vi "数据主动和反控发送.vi"() -> ()   [LabVIEW 2016, in "数据传输系统-04.lvlib"]
uses:
  <vilib>/ptbypt/NI_PtbyPt.lvlib
panel:
  in  "N个五分钟":u32
  out "QN":string
  out "元素":cluster{"命令编码CN":string, "QN":string}[](array[cluster])
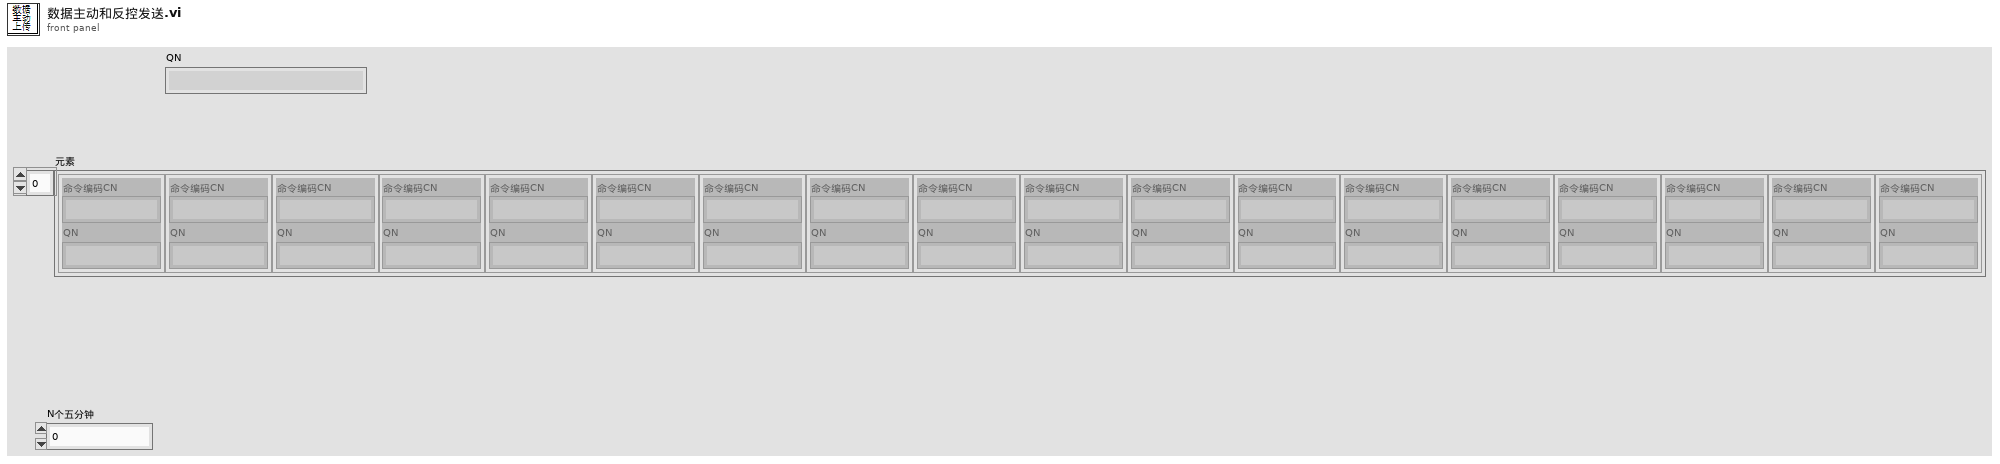
[diagram p1: front panel]
types:
  T1 = cluster{"setini":string, "sysini":string, "hechaini":string, "actualwrite":string, "actualread":string, "datasent":string, "反控命令信息队列":string, "反控与仪器交互":string}
  T2 = typedef "LVDateTimeRec.ctl" = cluster{"秒数的小数部分":dbl, "秒":i32, "分":i32, "时":i32, "日":i32, "月":i32, "年":i32, "天数（周）":i32, "天数（年）":i32, "DST":i32}
  T3 = enum16{"open", "replace", "create", "open or create", "replace or create", "replace or create with confirmation"}
  T4 = typedef "数据传输系统-04.lvlib/应用环境.ctl" = enum16{"STD", "GB212", "婉仪平台"}
  T5 = enum16{"关闭", "星期日", "星期一", "星期二", "星期三", "星期四", "星期五", "星期六"}
  T6 = enum16{"00点", "01点", "02点", "03点", "04点", "05点", "06点", "07点", "08点", "09点", "10点", "11点", "12点", "13点", "14点", "15点", "16点", "17点", "18点", "19点", "20点", "21点", "22点", "23点"}
  T7 = cluster{"[0]":string, "[1]":string, "[2]":string, "[3]":string, "[4]":string, "[5]":string, "[6]":string, "[7]":string, "[8]":string, "[9]":string, "[10]":string, "[11]":string, "[12]":string, "[13]":string, "[14]":string, "[15]":string, "[16]":string, "[17]":string, "[18]":string, "[19]":string, "[20]":string, "[21]":string, "[22]":string, "[23]":string, "[24]":string, "[25]":string, "[26]":string, "[27]":string, "[28]":string, "[29]":string, "[30]":string, "[31]":string, "[32]":string, "[33]":string, "[34]":string, "[35]":string, "[36]":string, "[37]":string, "[38]":string, "[39]":string, "[40]":string, "[41]":string, "[42]":string, "[43]":string, "[44]":string, "[45]":string, "[46]":string, "[47]":string, "[48]":string, "[49]":string, "[50]":string, "[51]":string, "[52]":string, "[53]":string, "[54]":string, "[55]":string, "[56]":string, "[57]":string, "[58]":string, "[59]":string, "[60]":string, "[61]":string, "[62]":string, "[63]":string, "[64]":string, "[65]":string, "[66]":string, "[67]":string, "[68]":string, "[69]":string, "[70]":string, "[71]":string, "[72]":string, "[73]":string, "[74]":string, "[75]":string}
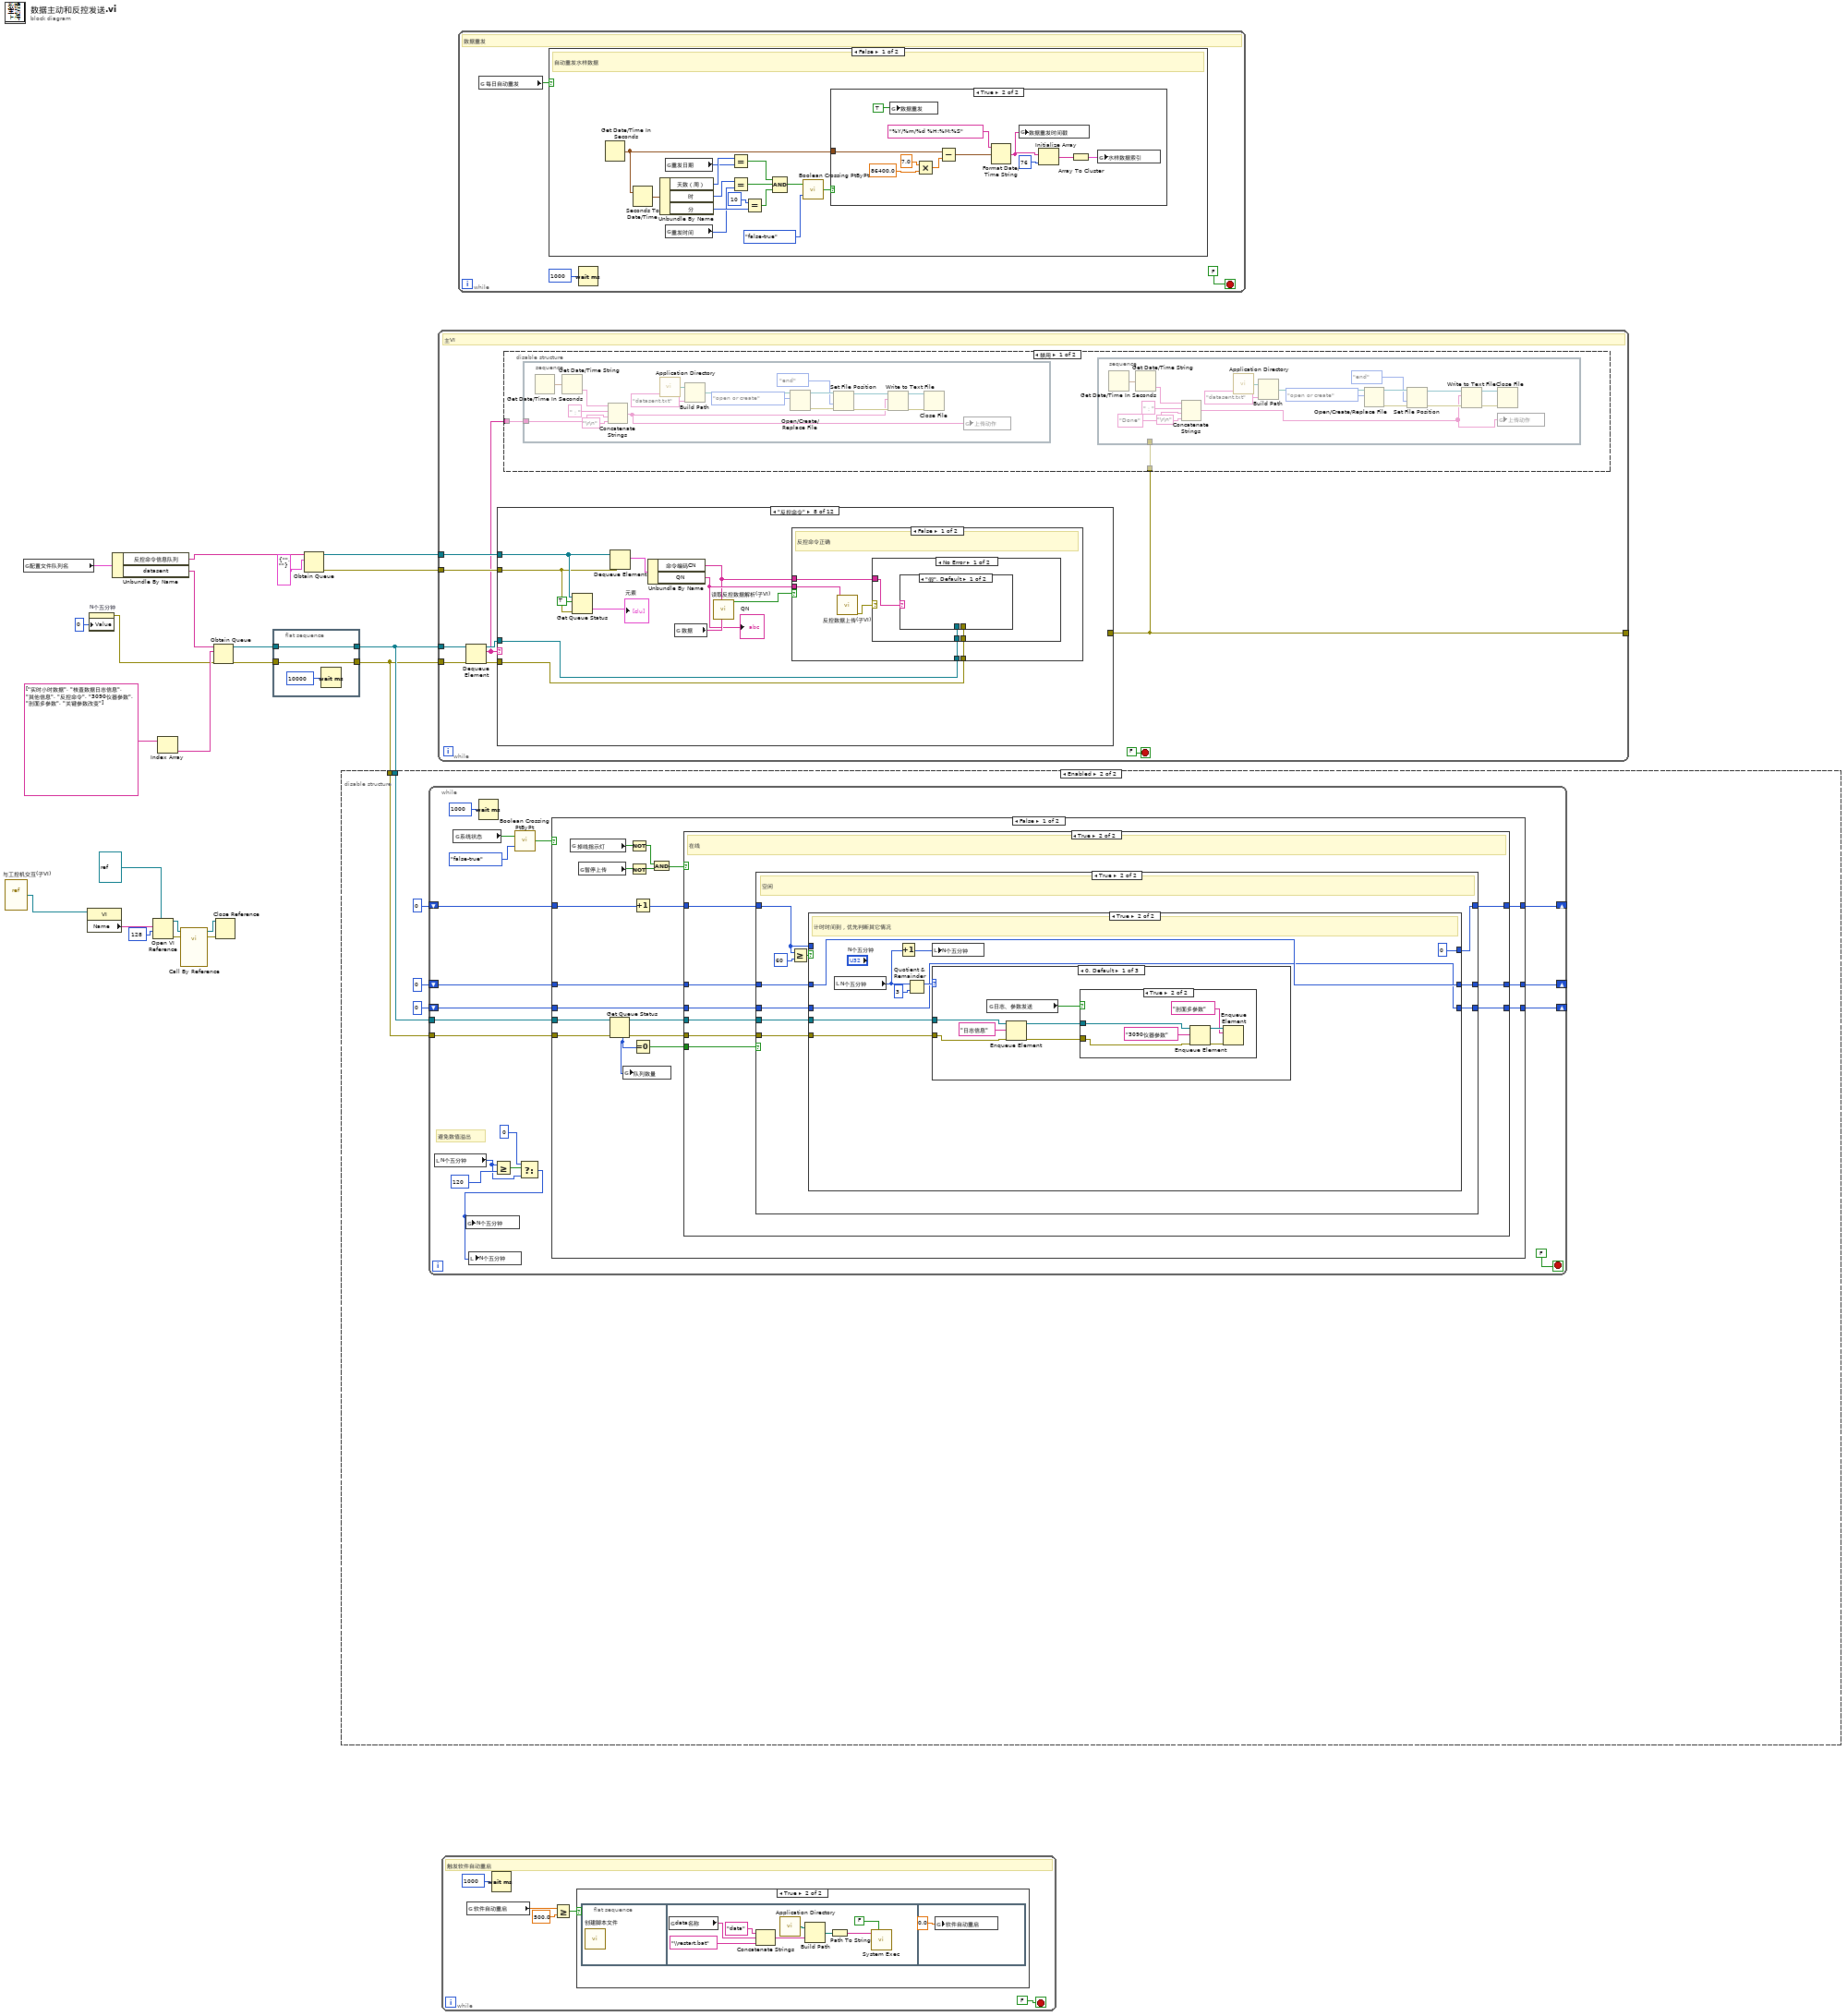
[diagram p0: block diagram]
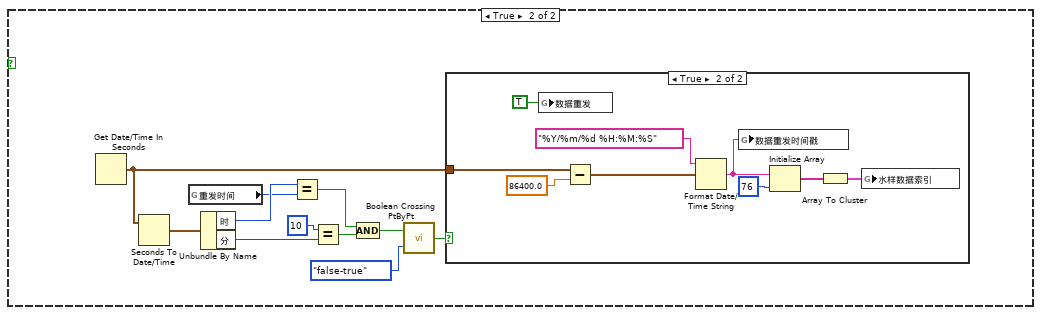
[diagram p3: hidden frame]
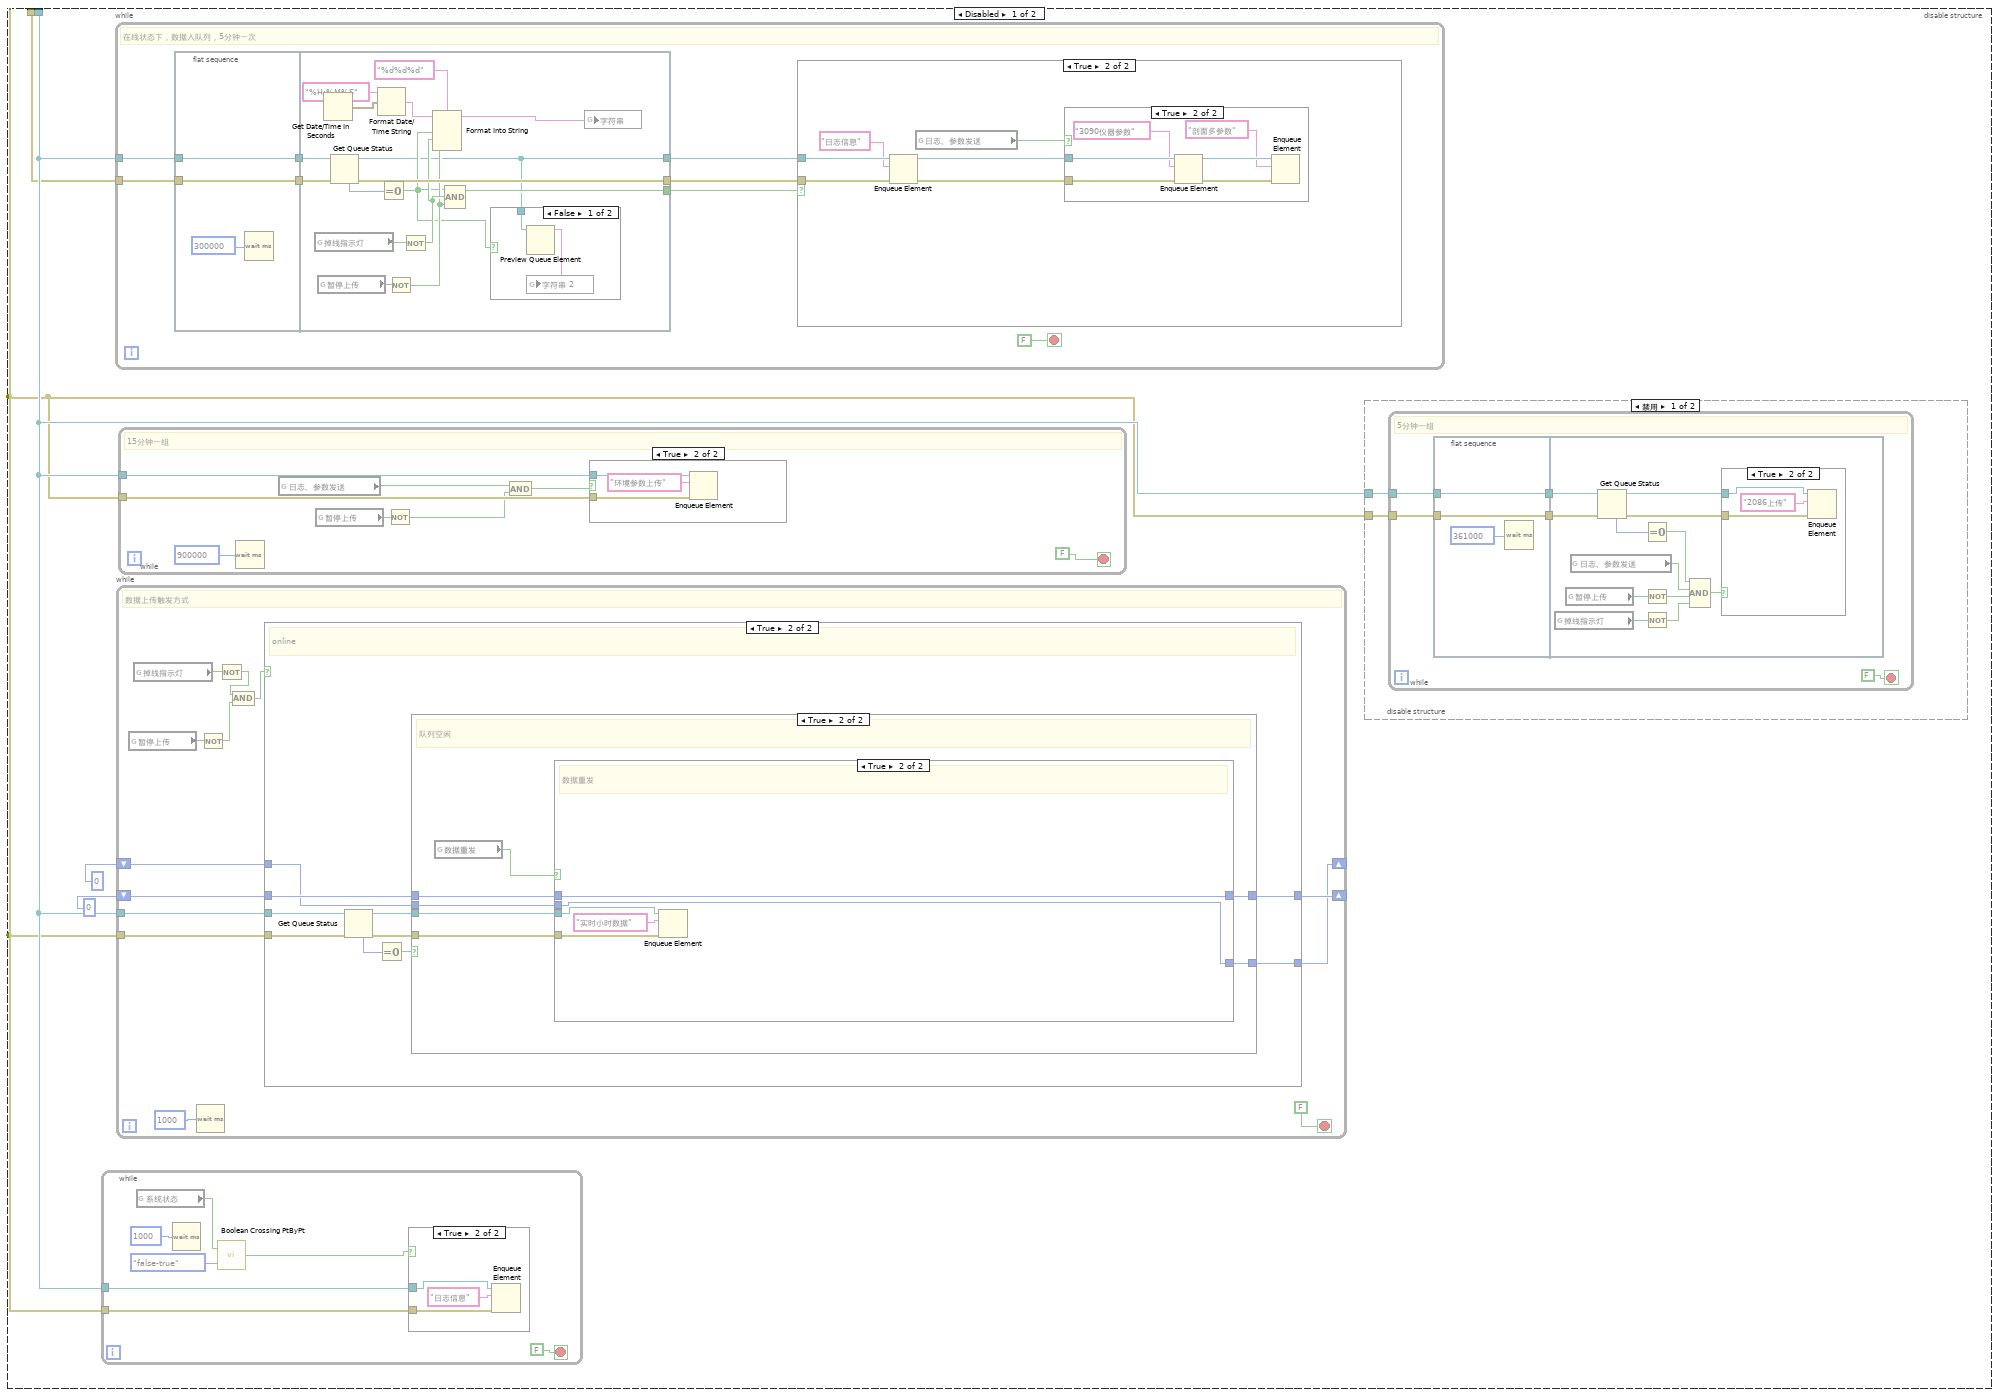
[diagram p5: hidden frame]
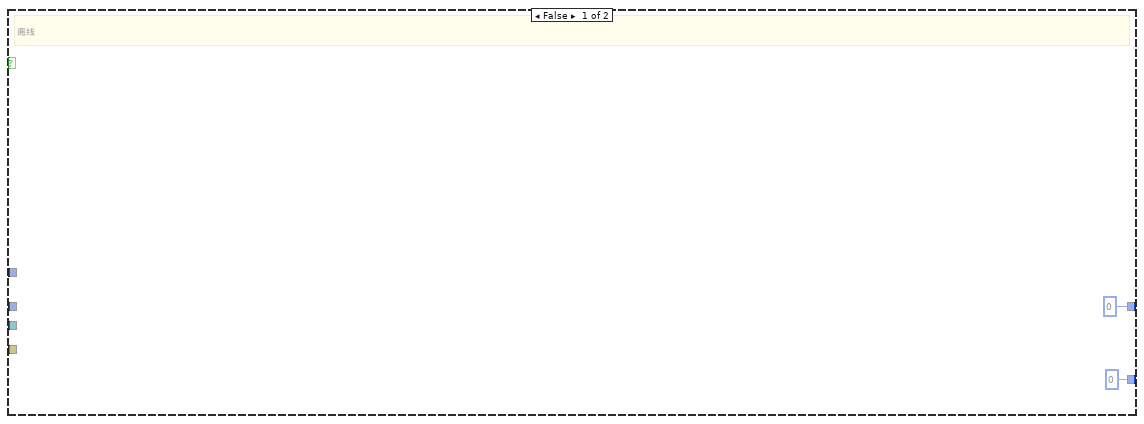
[diagram p9: hidden frame]
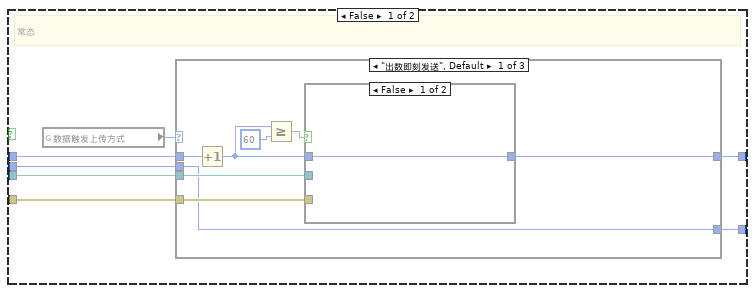
[diagram p11: hidden frame]
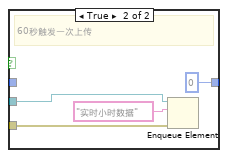
[diagram p12: hidden frame]
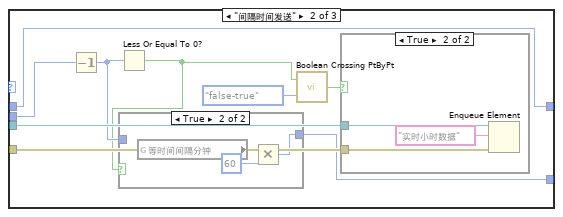
[diagram p13: hidden frame]
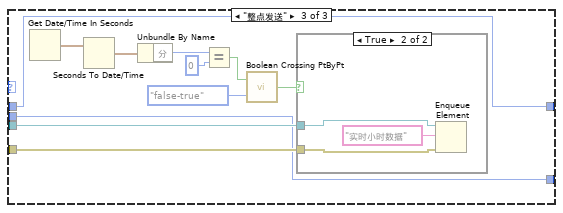
[diagram p16: hidden frame]
diagram:
  n1 = vi-ref "与工控机交互(子VI).vi"() -> (w15:refnum<vi>)
  n2 = global read "全局1.vi" "配置文件队列名"() -> (w5:T1)
  n3 = property class="VI"(reference=w15) -> ("Name"=w14:string)  [unwired: 1 in, 2 out]
  n4 = property on="N个五分钟" class="DigNum (strict)"("Value"=u32 0 ("N个五分钟")) -> (error out=w1:errorcluster)  [unwired: 2 in, 1 out]
  n5 = Unbundle By Name(w5) -> ("反控命令信息队列"=w9:string, "datasent"=w8:string)
  n6 = Open VI Reference(type specifier VI Refnum (for type only)=refnum<vi> refnum, vi path=w14, options=128 ("选项")) -> (vi reference=w12:refnum<vi>, error out=w6:errorcluster)  [unwired: 3 in]
  n7 = Index Array(array=string[] ["实时小时数据", "核查数据日志信息", "其他信息", "反控命令", "3090仪器参数", "剖面多参数", "关键参数改变"]) -> (element=w16:string)  [unwired: 1 in]
  n8 = call-by-ref "?"(reference=w12, error in=w6) -> (reference out=w10:refnum<vi>, error out=w7:errorcluster)  [unwired: 12 in]
  n9 = Obtain Queue(name (unnamed)=w8, element data type=w16, error in (no error)=w1) -> (queue out=w22:refnum<queue>, error out=w21:errorcluster)  [unwired: 2 in, 1 out]
  n10 = Close Reference(reference=w10, error in (no error)=w7) -> ()  [unwired: 1 out]
  n11 = flat-sequence {
    tunnel: w22 -> [w24]
    tunnel: [w24] -> w4
    tunnel: w21 -> [w23]
    tunnel: [w23] -> w3
    frame #0 {
      n12 = Wait (ms)(milliseconds to wait=u32 10000 ("等待时间（毫秒）")) -> ()  [unwired: 1 out]
    }
  }
  n13 = Obtain Queue(name (unnamed)=w9, element data type=cluster{"命令编码CN":string, "QN":string} {"命令编码CN"="", "QN"=""}) -> (queue out=w19:refnum<queue>, error out=w18:errorcluster)  [unwired: 3 in, 1 out]
  n14 = disable-structure shown="Enabled" {
    disable-tunnel: w4 -> [w27 w210]
    disable-tunnel: w3 -> [w26 w209]
    frame Disabled {
      n15 = while {
        tunnel: w27 -> [w57]
        tunnel: w26 -> [w56]
        stop <- FALSE stop-if-true
        n16 = global read "全局1.vi" "系统状态"() -> (w59:bool)
        n17 = Wait (ms)(milliseconds to wait=u32 1000 ("等待时间（毫秒）")) -> ()  [unwired: 1 out]
        n18 = call <vilib>:"Boolean Crossing PtByPt.vi"("direction"=enum16{"either", "false-true", "true-false"}."false-true", "input"=w59) -> ("crossing"=w55:bool)  [unwired: 1 in]
        n19 = case shown="True" w55 {
          tunnel: w57 -> [_ w62]
          tunnel: w56 -> [_ w63]
          frame False {
          }
          frame True {
            n20 = Enqueue Element(queue=w62, element="日志信息" ("元素"), error in (no error)=w63) -> ()  [unwired: 1 in, 3 out]
          }
        }
      }
      n21 = while {
        tunnel: w27 -> [w172]
        tunnel: w26 -> [w171]
        stop <- FALSE stop-if-true
        # "在线状态下，数据入队列，5分钟一次"
        n22 = flat-sequence {
          tunnel: w171 -> [w174]
          tunnel: w172 -> [w175]
          tunnel: [w175] -> w166
          tunnel: [w174] -> w165
          tunnel: [w177] -> w170
          tunnel: [w189] -> w169
          tunnel: [w187] -> w167
          tunnel: w166 -> [w191]
          tunnel: w165 -> [w190]
          frame #0 {
            n23 = Wait (ms)(milliseconds to wait=u32 300000 ("等待时间（毫秒）")) -> ()  [unwired: 1 out]
          }
          frame #1 {
            n24 = global read "全局 数据发送重叠.vi" "掉线指示灯"() -> (w188:bool)
            n25 = global read "断电保存全局.vi" "暂停上传"() -> (w186:bool)
            n26 = Get Date/Time In Seconds() -> (seconds since 1Jan1904=w184:timestamp)
            n27 = Get Queue Status(queue=w191, error in (no error)=w190) -> (queue out=w177:refnum<queue>, error out=w189:errorcluster, # elements in queue=w185:i32)  [unwired: 1 in, 5 out]
            n28 = Format Date/Time String(time format string (%c)="%H:%M%S" ("时间格式字符串(%c)"), seconds (now)=w184) -> (date/time string=w182:string)  [unwired: 1 in]
            n29 = Equal To 0?(x=w185) -> (x = 0?=w178:bool)
            n30 = Not(x=w186) -> (.not. x?=w179:bool)
            n31 = Not(x=w188) -> (.not. x?=w180:bool)
            n32 = Format Into String(format string="%d%d%d" ("格式字符串"), initial string=w182, w178, w180, w179) -> (resulting string=w176:string)  [unwired: 1 in, 1 out]
            n33 = Compound Arithmetic op=AND ("复合运算")(w178, w180, w179) -> (w187:bool)
            n34 = case shown="False" w178 {
              tunnel: w177 -> [w193 _]
              frame False {
                n35 = Preview Queue Element(queue=w193) -> (element=w192:string)  [unwired: 2 in, 3 out]
                n36 = global write "全局 水样时间.vi" "字符串 2"(w192) -> ()
              }
              frame True {
              }
            }
            n37 = global write "全局 水样时间.vi" "字符串"(w176) -> ()
          }
        }
        n38 = case shown="True" w167 {
          tunnel: w170 -> [_ w199]
          tunnel: w169 -> [_ w198]
          frame False {
          }
          frame True {
            n39 = Enqueue Element(queue=w199, element="日志信息" ("元素"), error in (no error)=w198) -> (queue out=w196:refnum<queue>, error out=w195:errorcluster)  [unwired: 1 in, 1 out]
            n40 = global read "断电保存全局.vi" "日志、参数发送"() -> (w194:bool)
            n41 = case shown="True" w194 {
              tunnel: w196 -> [_ w205]
              tunnel: w195 -> [_ w204]
              frame False {
              }
              frame True {
                n42 = Enqueue Element(queue=w205, element="3090仪器参数" ("元素"), error in (no error)=w204) -> (queue out=w202:refnum<queue>, error out=w201:errorcluster)  [unwired: 1 in, 1 out]
                n43 = Enqueue Element(queue=w202, element="剖面多参数" ("元素"), error in (no error)=w201) -> ()  [unwired: 1 in, 3 out]
              }
            }
          }
        }
      }
      n44 = while {
        tunnel: w27 -> [w72]
        tunnel: w26 -> [w71]
        shift-right: [w74] -> _
        shift-left: 0 -> [w75]
        shift-right: [w65] -> _
        shift-left: 0 -> [w66]
        stop <- FALSE stop-if-true
        # "数据上传触发方式"
        n45 = global read "断电保存全局.vi" "暂停上传"() -> (w69:bool)
        n46 = global read "全局 数据发送重叠.vi" "掉线指示灯"() -> (w76:bool)
        n47 = Wait (ms)(milliseconds to wait=u32 1000 ("等待时间（毫秒）")) -> ()  [unwired: 1 out]
        n48 = Not(x=w69) -> (.not. x?=w68:bool)
        n49 = Not(x=w76) -> (.not. x?=w70:bool)
        n50 = And(x=w70, y=w68) -> (x .and. y?=w67:bool)
        n51 = case shown="True" w67 {
          tunnel: w75 -> [_ w89]
          tunnel: [0 w88] -> w74
          tunnel: w72 -> [_ w86]
          tunnel: w71 -> [_ w85]
          tunnel: w66 -> [_ w81]
          tunnel: [0 w80] -> w65
          frame False {
            # "离线"
          }
          frame True {
            # "online"
            n52 = Get Queue Status(queue=w86, error in (no error)=w85) -> (queue out=w83:refnum<queue>, error out=w82:errorcluster, # elements in queue=w87:i32)  [unwired: 1 in, 5 out]
            n53 = Equal To 0?(x=w87) -> (x = 0?=w84:bool)
            n54 = case shown="True" w84 {
              tunnel: w83 -> [_ w98]
              tunnel: w82 -> [_ w97]
              tunnel: w89 -> [w91 w96]
              tunnel: [w91 w95] -> w88
              tunnel: w81 -> [w90 w94]
              tunnel: [w90 w93] -> w80
              frame False {
                # "队列忙碌中"
              }
              frame True {
                # "队列空闲"
                n55 = global read "断电保存全局.vi" "数据重发"() -> (w92:bool)
                n56 = case shown="True" w92 {
                  tunnel: w98 -> [w105 w152]
                  tunnel: w97 -> [w104 w151]
                  tunnel: w96 -> [w102 w150]
                  tunnel: [w101 w150] -> w95
                  tunnel: w94 -> [w100 w149]
                  tunnel: [w99 w149] -> w93
                  frame False {
                    # "常态"
                    n57 = global read "断电保存全局.vi" "数据触发上传方式"() -> (w103:enum16{"出数即刻发送", "间隔时间发送", "整点发送"})
                    n58 = case shown="\"出数即刻发送\", Default" w103 {
                      tunnel: w105 -> [w108 w126 w139]
                      tunnel: w104 -> [w107 w125 w138]
                      tunnel: w102 -> [w113 w127 w137]
                      tunnel: [w109 w127 w137] -> w101
                      tunnel: w100 -> [w106 w122 w135]
                      tunnel: [w106 w121 w135] -> w99
                      frame "出数即刻发送", Default {
                        n59 = Increment(x=w113) -> (x+1=w110:i32)
                        n60 = Greater Or Equal?(x=w110, y=60) -> (x >= y?=w111:bool)
                        n61 = case shown="False" w111 {
                          tunnel: w110 -> [w114 _]
                          tunnel: [w114 0] -> w109
                          tunnel: w108 -> [_ w116]
                          tunnel: w107 -> [_ w115]
                          frame False {
                          }
                          frame True {
                            # "60秒触发一次上传"
                            n62 = Enqueue Element(queue=w116, element="实时小时数据" ("元素"), error in (no error)=w115) -> ()  [unwired: 1 in, 3 out]
                          }
                        }
                      }
                      frame "间隔时间发送" {
                        n63 = Decrement(x=w122) -> (x-1=w120:i32)
                        n64 = Less Or Equal To 0?(x=w120) -> (x <= 0?=w119:bool)
                        n65 = case shown="True" w119 {
                          tunnel: w120 -> [w128 _]
                          tunnel: [w128 w129] -> w121
                          frame False {
                          }
                          frame True {
                            n66 = global read "断电保存全局.vi" "等时间间隔分钟"() -> (w130:i32)
                            n67 = Multiply(x=w130, y=60) -> (x*y=w129:i32)
                          }
                        }
                        n68 = call <vilib>:"Boolean Crossing PtByPt.vi"("direction"=enum16{"either", "false-true", "true-false"}."false-true", "input"=w119) -> ("crossing"=w123:bool)  [unwired: 1 in]
                        n69 = case shown="True" w123 {
                          tunnel: w126 -> [_ w133]
                          tunnel: w125 -> [_ w132]
                          frame False {
                          }
                          frame True {
                            n70 = Enqueue Element(queue=w133, element="实时小时数据" ("元素"), error in (no error)=w132) -> ()  [unwired: 1 in, 3 out]
                          }
                        }
                      }
                      frame "整点发送" {
                        n71 = Get Date/Time In Seconds() -> (seconds since 1Jan1904=w144:timestamp)
                        n72 = Seconds To Date/Time(time stamp (now)=w144) -> (date time rec=w145:T2)  [unwired: 1 in]
                        n73 = Unbundle By Name(w145) -> ("分"=w143:i32)
                        n74 = Equal?(x=w143, y=0) -> (x = y?=w141:bool)
                        n75 = call <vilib>:"Boolean Crossing PtByPt.vi"("direction"=enum16{"either", "false-true", "true-false"}."false-true", "input"=w141) -> ("crossing"=w136:bool)  [unwired: 1 in]
                        n76 = case shown="True" w136 {
                          tunnel: w139 -> [_ w147]
                          tunnel: w138 -> [_ w146]
                          frame False {
                          }
                          frame True {
                            n77 = Enqueue Element(queue=w147, element="实时小时数据" ("元素"), error in (no error)=w146) -> ()  [unwired: 1 in, 3 out]
                          }
                        }
                      }
                    }
                  }
                  frame True {
                    # "数据重发"
                    n78 = Enqueue Element(queue=w152, element="实时小时数据" ("元素"), error in (no error)=w151) -> ()  [unwired: 1 in, 3 out]
                  }
                }
              }
            }
          }
        }
      }
      n79 = while {
        tunnel: w27 -> [w159]
        tunnel: w26 -> [w158]
        stop <- FALSE stop-if-true
        # "15分钟一组"
        n80 = Wait (ms)(milliseconds to wait=u32 900000 ("等待时间（毫秒）")) -> ()  [unwired: 1 out]
        n81 = global read "断电保存全局.vi" "日志、参数发送"() -> (w156:bool)
        n82 = global read "断电保存全局.vi" "暂停上传"() -> (w157:bool)
        n83 = Not(x=w157) -> (.not. x?=w155:bool)
        n84 = And(x=w156, y=w155) -> (x .and. y?=w154:bool)
        n85 = case shown="True" w154 {
          tunnel: w159 -> [_ w163]
          tunnel: w158 -> [_ w162]
          frame False {
          }
          frame True {
            n86 = Enqueue Element(queue=w163, element="环境参数上传" ("元素"), error in (no error)=w162) -> ()  [unwired: 1 in, 3 out]
          }
        }
      }
      n87 = disable-structure shown="禁用" {
        disable-tunnel: w27 -> [w31 _]
        disable-tunnel: w26 -> [w30 _]
        frame Disabled {
          n88 = while {
            tunnel: w31 -> [w35]
            tunnel: w30 -> [w34]
            stop <- FALSE stop-if-true
            # "5分钟一组"
            n89 = flat-sequence {
              tunnel: w34 -> [w38]
              tunnel: w35 -> [w39]
              tunnel: [w39] -> w33
              tunnel: [w38] -> w32
              tunnel: w33 -> [w46]
              tunnel: w32 -> [w45]
              frame #0 {
                n90 = Wait (ms)(milliseconds to wait=u32 361000 ("等待时间（毫秒）")) -> ()  [unwired: 1 out]
              }
              frame #1 {
                n91 = global read "全局 数据发送重叠.vi" "掉线指示灯"() -> (w43:bool)
                n92 = global read "断电保存全局.vi" "暂停上传"() -> (w51:bool)
                n93 = global read "断电保存全局.vi" "日志、参数发送"() -> (w50:bool)
                n94 = Get Queue Status(queue=w46, error in (no error)=w45) -> (queue out=w44:refnum<queue>, error out=w40:errorcluster, # elements in queue=w47:i32)  [unwired: 1 in, 5 out]
                n95 = Equal To 0?(x=w47) -> (x = 0?=w41:bool)
                n96 = Not(x=w51) -> (.not. x?=w49:bool)
                n97 = Not(x=w43) -> (.not. x?=w42:bool)
                n98 = Compound Arithmetic op=AND ("复合运算")(w41, w50, w49, w42) -> (w48:bool)
                n99 = case shown="True" w48 {
                  tunnel: w44 -> [_ w53]
                  tunnel: w40 -> [_ w52]
                  frame False {
                  }
                  frame True {
                    n100 = Enqueue Element(queue=w53, element="2086上传" ("元素"), error in (no error)=w52) -> ()  [unwired: 1 in, 3 out]
                  }
                }
              }
            }
          }
        }
        frame Enabled {
        }
      }
    }
    frame Enabled {
      n101 = while {
        tunnel: w210 -> [w223]
        tunnel: w209 -> [w222]
        shift-right: [w221] -> _
        shift-left: 0 -> [w216]
        shift-right: [w220] -> _
        shift-left: 0 -> [w217]
        shift-right: [w219] -> _
        shift-left: 0 -> [w218]
        stop <- FALSE stop-if-true
        # "避免数值溢出"
        n102 = local read "N个五分钟"() -> (w212:u32)
        n103 = global read "全局1.vi" "系统状态"() -> (w226:bool)
        n104 = Wait (ms)(milliseconds to wait=u32 1000 ("等待时间（毫秒）")) -> ()  [unwired: 1 out]
        n105 = Greater Or Equal?(x=w212, y=u32 120) -> (x >= y?=w214:bool)
        n106 = call <vilib>:"Boolean Crossing PtByPt.vi"("direction"=enum16{"either", "false-true", "true-false"}."false-true", "input"=w226) -> ("crossing"=w224:bool)  [unwired: 1 in]
        n107 = Select(t=u32 0 ("y"), s=w214, f=w212) -> (s? t:f=w211:u32)
        n108 = global write "全局 水样时间.vi" "N个五分钟"(w211) -> ()
        n109 = local write "N个五分钟"(w211) -> ()
        n110 = case shown="False" w224 {
          tunnel: w223 -> [w234 w369]
          tunnel: w222 -> [w233 w370]
          tunnel: [w241 w368] -> w221
          tunnel: [w240 w367] -> w220
          tunnel: w216 -> [w239 w368]
          tunnel: w217 -> [w238 w367]
          tunnel: w218 -> [w237 w366]
          tunnel: [w235 w366] -> w219
          frame False {
            n111 = global read "全局 数据发送重叠.vi" "掉线指示灯"() -> (w246:bool)
            n112 = global read "断电保存全局.vi" "暂停上传"() -> (w244:bool)
            n113 = Get Queue Status(queue=w234, error in (no error)=w233) -> (queue out=w232:refnum<queue>, error out=w231:errorcluster, # elements in queue=w229:i32)  [unwired: 1 in, 5 out]
            n114 = global write "全局 水样时间.vi" "队列数量"(w229) -> ()
            n115 = Not(x=w246) -> (.not. x?=w245:bool)
            n116 = Not(x=w244) -> (.not. x?=w243:bool)
            n117 = Increment(x=w237) -> (x+1=w236:i32)
            n118 = Equal To 0?(x=w229) -> (x = 0?=w230:bool)
            n119 = And(x=w245, y=w243) -> (x .and. y?=w242:bool)
            n120 = case shown="True" w242 {
              tunnel: [w247 w255] -> w241
              tunnel: [w247 w253] -> w240
              tunnel: w232 -> [_ w250]
              tunnel: w239 -> [_ w256]
              tunnel: w238 -> [_ w254]
              tunnel: w236 -> [_ w252]
              tunnel: [w247 w251] -> w235
              tunnel: w231 -> [_ w249]
              tunnel: w230 -> [_ w248]
              frame False {
                w247 = 0
                # "离线状态"
              }
              frame True {
                # "在线"
                n121 = case shown="True" w248 {
                  tunnel: w256 -> [w259 w265]
                  tunnel: [w259 w264] -> w255
                  tunnel: w254 -> [w258 w267]
                  tunnel: [w258 w266] -> w253
                  tunnel: w250 -> [_ w269]
                  tunnel: w249 -> [_ w268]
                  tunnel: w252 -> [w257 w260]
                  tunnel: [w257 w261] -> w251
                  frame False {
                    # "忙碌"
                  }
                  frame True {
                    # "空闲"
                    n122 = Greater Or Equal?(x=w260, y=60) -> (x >= y?=w262:bool)
                    n123 = case shown="True" w262 {
                      tunnel: w269 -> [w279 w340]
                      tunnel: w268 -> [w278 w339]
                      tunnel: w267 -> [w277 w346]
                      tunnel: [w276 w346] -> w266
                      tunnel: w265 -> [w275 w338]
                      tunnel: [w274 w338] -> w264
                      tunnel: [w273 0] -> w261
                      tunnel: w260 -> [w273 _]
                      frame False {
                        # "五分钟计时未到"
                        n124 = global read "断电保存全局.vi" "数据重发"() -> (w272:bool)
                        n125 = call <vilib>:"Boolean Crossing PtByPt.vi"("direction"=enum16{"either", "false-true", "true-false"}."false-true", "input"=w272) -> ("crossing"=w270:bool)  [unwired: 1 in]
                        n126 = case shown="True" w272 {
                          tunnel: w279 -> [w284 w334]
                          tunnel: w278 -> [w283 w333]
                          tunnel: w277 -> [w285 w331]
                          tunnel: [w282 w331] -> w276
                          tunnel: w275 -> [w280 w332]
                          tunnel: [w281 w332] -> w274
                          tunnel: w270 -> [_ w330]
                          frame False {
                            n127 = global read "断电保存全局.vi" "数据触发上传方式"() -> (w286:enum16{"出数即刻发送", "间隔时间发送", "整点发送"})
                            n128 = case shown="\"整点发送\"" w286 {
                              tunnel: w285 -> [w294 w300 w316]
                              tunnel: w284 -> [w291 w303 w319]
                              tunnel: w283 -> [w290 w302 w318]
                              tunnel: [w289 w300 w316] -> w282
                              tunnel: w280 -> [w288 w307 w317]
                              tunnel: [w288 w301 w317] -> w281
                              frame "出数即刻发送", Default {
                                n129 = Increment(x=w294) -> (x+1=w287:i32)
                                n130 = Greater Or Equal?(x=w287, y=30) -> (x >= y?=w292:bool)
                                n131 = case shown="True" w292 {
                                tunnel: w291 -> [_ w299]
                                tunnel: w290 -> [_ w298]
                                tunnel: [w295 0] -> w289
                                tunnel: w287 -> [w295 _]
                                frame False {
                                }
                                frame True {
                                n132 = Enqueue Element(queue=w299, element="实时小时数据", error in (no error)=w298) -> ()  [unwired: 1 in, 3 out]
                                }
                                }
                              }
                              frame "间隔时间发送" {
                                n133 = Decrement(x=w307) -> (x-1=w306:i32)
                                n134 = Less Or Equal To 0?(x=w306) -> (x <= 0?=w305:bool)
                                n135 = case shown="True" w305 {
                                tunnel: w306 -> [w312 _]
                                tunnel: [w312 w313] -> w301
                                frame False {
                                }
                                frame True {
                                n136 = global read "断电保存全局.vi" "等时间间隔分钟"() -> (w314:i32)
                                n137 = Multiply(x=w314, y=60) -> (x*y=w313:i32)
                                }
                                }
                                n138 = call <vilib>:"Boolean Crossing PtByPt.vi"("direction"=enum16{"either", "false-true", "true-false"}."false-true", "input"=w305) -> ("crossing"=w304:bool)  [unwired: 1 in]
                                n139 = case shown="True" w304 {
                                tunnel: w303 -> [_ w310]
                                tunnel: w302 -> [_ w309]
                                frame False {
                                }
                                frame True {
                                n140 = Enqueue Element(queue=w310, element="实时小时数据" ("元素"), error in (no error)=w309) -> ()  [unwired: 1 in, 3 out]
                                }
                                }
                              }
                              frame "整点发送" {
                                n141 = Get Date/Time In Seconds() -> (seconds since 1Jan1904=w322:timestamp)
                                n142 = Seconds To Date/Time(time stamp (now)=w322) -> (date time rec=w321:T2)  [unwired: 1 in]
                                n143 = Unbundle By Name(w321) -> ("分"=w323:i32)
                                n144 = Equal?(x=w323, y=0) -> (x = y?=w325:bool)
                                n145 = call <vilib>:"Boolean Crossing PtByPt.vi"("direction"=enum16{"either", "false-true", "true-false"}."false-true", "input"=w325) -> ("crossing"=w320:bool)  [unwired: 1 in]
                                n146 = case shown="True" w320 {
                                tunnel: w319 -> [_ w328]
                                tunnel: w318 -> [_ w327]
                                frame False {
                                }
                                frame True {
                                n147 = Enqueue Element(queue=w328, element="实时小时数据" ("元素"), error in (no error)=w327) -> ()  [unwired: 1 in, 3 out]
                                }
                                }
                              }
                            }
                          }
                          frame True {
                            n148 = case shown="True" w330 {
                              tunnel: w334 -> [_ w337]
                              tunnel: w333 -> [_ w336]
                              frame False {
                              }
                              frame True {
                                n149 = Enqueue Element(queue=w337, element="实时小时数据" ("元素"), error in (no error)=w336) -> ()  [unwired: 1 in, 3 out]
                              }
                            }
                          }
                        }
                      }
                      frame True {
                        # "计时时间到，优先判断其它情况"
                        n150 = local read "N个五分钟"() -> (w341:u32)
                        n151 = Increment(x=w341) -> (x+1=w342:u32)
                        n152 = Quotient & Remainder(x=w341, y=u32 3) -> (x-y*floor(x/y)=w343:u32)  [unwired: 1 out]
                        n153 = local write "N个五分钟"(w342) -> ()
                        n154 = case shown="0, Default" w343 {
                          tunnel: w340 -> [w348 w361 w363]
                          tunnel: w339 -> [w347 w360 w364]
                          frame 0, Default {
                            n155 = global read "断电保存全局.vi" "日志、参数发送"() -> (w352:bool)
                            n156 = Enqueue Element(queue=w348, element="日志信息" ("元素"), error in (no error)=w347) -> (queue out=w350:refnum<queue>, error out=w351:errorcluster)  [unwired: 1 in, 1 out]
                            n157 = case shown="True" w352 {
                              tunnel: w350 -> [_ w358]
                              tunnel: w351 -> [_ w357]
                              frame False {
                              }
                              frame True {
                                n158 = Enqueue Element(queue=w358, element="3090仪器参数" ("元素"), error in (no error)=w357) -> (queue out=w355:refnum<queue>, error out=w354:errorcluster)  [unwired: 1 in, 1 out]
                                n159 = Enqueue Element(queue=w355, element="剖面多参数" ("元素"), error in (no error)=w354) -> ()  [unwired: 1 in, 3 out]
                              }
                            }
                          }
                          frame 1 {
                            n160 = Enqueue Element(queue=w361, element="2086上传" ("元素"), error in (no error)=w360) -> ()  [unwired: 1 in, 3 out]
                            n161 = global write "全局1.vi" "2086上传"(TRUE ("2086上传")) -> ()
                          }
                          frame 2 {
                            n162 = Enqueue Element(queue=w363, element="环境参数上传" ("元素"), error in (no error)=w364) -> ()  [unwired: 1 in, 3 out]
                          }
                        }
                      }
                    }
                  }
                }
              }
            }
          }
          frame True {
            n163 = Enqueue Element(queue=w369, element="日志信息" ("元素"), error in (no error)=w370) -> ()  [unwired: 1 in, 3 out]
          }
        }
      }
    }
  }
  n164 = while {
    tunnel: w4 -> [w375]
    tunnel: w3 -> [w374]
    tunnel: w19 -> [w377]
    tunnel: w18 -> [w376]
    tunnel: [w372] -> _
    stop <- FALSE stop-if-true
    # "主VI"
    n165 = Dequeue Element(queue=w375, error in (no error)=w374) -> (queue out=w379:refnum<queue>, element=w373:string, error out=w378:errorcluster)  [unwired: 1 in, 1 out]
    n166 = case shown="\"反控命令\"" w373 {
      tunnel: w379 -> [_ _ w423 _ _ _ _ w445 _ _ _ _]
      tunnel: w378 -> [_ _ _ _ _ _ _ w444 _ _ _ _]
      tunnel: w377 -> [_ _ _ _ _ _ _ w452 _ _ _ _]
      tunnel: w376 -> [_ _ _ _ _ _ _ w451 _ _ _ _]
      tunnel: [_ w417 w422 w429 w435 w440 _ _ w465 w471 w479 _] -> w372
      frame Default {
      }
      frame "实时小时数据" {
        n167 = call "变量初始化.vi"() -> ("错误输出"=w418:errorcluster)  [unwired: 11 in]
        n168 = call "实时小时数据单参数上传.vi"("错误输入（无错误）"=w418) -> ("数据发送起始时间"=w420:timestamp, "error out"=w419:errorcluster)  [unwired: 13 in]
        n169 = global write "全局1.vi" "数据发送起始时间"(w420) -> ()
        n170 = call <vilib>:"Clear Errors.vi"("error in (no error)"=w419) -> ("error out"=w417:errorcluster)  [unwired: 5 in, 1 out]
      }
      frame "日志信息" {
        n171 = call "日志信息出发送队列 (子VI).vi"("queue out"=w423) -> ("错误输出"=w421:errorcluster)  [unwired: 10 in]
        n172 = call <vilib>:"Clear Errors.vi"("error in (no error)"=w421) -> ("error out"=w422:errorcluster)  [unwired: 5 in, 1 out]
      }
      frame "关键参数改变" {
        n173 = global read "断电保存全局.vi" "仪器参数发送"() -> (w427:bool)
        n174 = global read "断电保存全局.vi" "应用环境"() -> (w428:T4)
        n175 = Equal?(x=w428, y=应用环境."STD" ("应用环境")) -> (x = y?=w426:bool)
        n176 = And(x=w427, y=w426) -> (x .and. y?=w425:bool)
        n177 = case shown="True" w425 {
          tunnel: [_ w430] -> w429
          frame False {
          }
          frame True {
            n178 = call "仪器参数改变发送 (子VI).vi"() -> ("错误输出"=w431:errorcluster)  [unwired: 11 in]
            n179 = call "采配水仪器参数改变发送 (子VI).vi"("错误输入"=w431) -> ("错误输出"=w430:errorcluster)  [unwired: 10 in]
          }
        }
      }
      frame "校准信息改变" {
        n180 = global read "断电保存全局.vi" "应用环境"() -> (w434:T4)
        n181 = Equal?(x=w434, y=应用环境."STD" ("应用环境")) -> (x = y?=w433:bool)
        n182 = case shown="True" w433 {
          tunnel: [_ w436] -> w435
          frame False {
          }
          frame True {
            n183 = call "校准信息改变发送 (子VI).vi"() -> ("错误输出"=w436:errorcluster)  [unwired: 11 in]
          }
        }
      }
      frame "3201告警信息改变" {
        n184 = global read "断电保存全局.vi" "应用环境"() -> (w439:T4)
        n185 = Equal?(x=w439, y=应用环境."婉仪平台") -> (x = y?=w438:bool)
        n186 = case shown="True" w438 {
          tunnel: [_ w441] -> w440
          frame False {
          }
          frame True {
            n187 = call "3201告警信息改变发送 (子VI).vi"() -> ("错误输出"=w441:errorcluster)  [unwired: 11 in]
          }
        }
      }
      frame "其他信息" {
      }
      frame "反控命令" {
        n188 = Get Queue Status(queue=w452, return elements? (F)=TRUE ("返回元素？(F)"), error in (no error)=w451) -> (elements=→"元素":cluster{"命令编码CN":string, "QN":string}[])  [unwired: 7 out]
        n189 = Dequeue Element(queue=w452, error in (no error)=w451) -> (element=w448:cluster{"命令编码CN":string, "QN":string})  [unwired: 1 in, 3 out]
        n190 = Unbundle By Name(w448) -> ("命令编码CN"=w442:string, "QN"=w443:string)
        "QN" <- w443
        n191 = global read "全局1.vi" "数据"() -> (w450:string)
        n192 = call "读取反控数据解析(子VI).vi"("数据"=w450, "命令编码CN"=w442) -> ("反控命令错误？"=w449:bool)  [unwired: 8 in, 1 out]
        n193 = case shown="False" w449 {
          tunnel: w443 -> [w457 _]
          tunnel: w445 -> [w455 _]
          tunnel: w444 -> [w454 _]
          tunnel: w442 -> [w453 _]
          frame False {
            # "反控命令正确"
            n194 = call "反控数据上传(子VI).vi"("QN"=w457) -> ("error out"=w456:errorcluster)  [unwired: 10 in]
            n195 = case shown="No Error" w456 {
              tunnel: w455 -> [w460 _]
              tunnel: w454 -> [w459 _]
              tunnel: w453 -> [w458 _]
              frame No Error {
                n196 = case shown="\"假\", Default" w458 {
                  tunnel: w460 -> [_ w463]
                  tunnel: w459 -> [_ w462]
                  frame "假", Default {
                  }
                  frame "2084", "3056" {
                    n197 = Enqueue Element(queue=w463, element="日志信息" ("元素"), error in (no error)=w462) -> ()  [unwired: 1 in, 3 out]
                  }
                }
              }
              frame Error {
              }
            }
          }
          frame True {
            # "反控命令错误"
          }
        }
      }
      frame "3090仪器参数" {
        n198 = global read "断电保存全局.vi" "应用环境"() -> (w464:T4)
        n199 = case shown="\"STD\"" w464 {
          tunnel: [w466 _] -> w465
          frame "STD" {
            n200 = call "3090仪器参数上传.vi"() -> ("error out"=w467:errorcluster)  [unwired: 15 in]
            n201 = call "变量初始化.vi"("错误输入（无错误）"=w467) -> ("错误输出"=w466:errorcluster)  [unwired: 10 in]
          }
          frame "GB212", Default {
          }
        }
      }
      frame "剖面多参数" {
        n202 = global read "断电保存全局.vi" "应用环境"() -> (w470:T4)
        n203 = call "剖面多参数上传.vi"() -> ("error out"=w469:errorcluster)  [unwired: 15 in]
        n204 = call <vilib>:"Clear Errors.vi"("error in (no error)"=w469) -> ("error out"=w468:errorcluster)  [unwired: 5 in, 1 out]
        n205 = case shown="\"STD\"" w470 {
          tunnel: [w474 w475 w478] -> w471
          tunnel: w468 -> [w473 w475 w477]
          frame "STD" {
            n206 = call "海流计数据上传.vi"("错误输入（无错误）"=w473) -> ("error out"=w472:errorcluster)  [unwired: 10 in]
            n207 = call "新剖面数据上传.vi"("错误输入（无错误）"=w472) -> ("error out"=w474:errorcluster)  [unwired: 14 in]
          }
          frame "GB212", Default {
            n208 = global write "断电保存全局.vi" "剖面数据重发"(FALSE ("剖面数据重发")) -> ()
          }
          frame "婉仪平台" {
            n209 = call "新剖面数据上传.vi"("错误输入（无错误）"=w477) -> ("error out"=w478:errorcluster)  [unwired: 14 in]
          }
        }
      }
      frame "环境参数上传" {
        n210 = call "环境参数上传.vi"() -> ("error out"=w479:errorcluster)  [unwired: 15 in]
      }
      frame "2086上传" {
        n211 = flat-sequence {
          frame #0 {
            n212 = call "2086发送.vi"() -> ()  [unwired: 12 in]
          }
          frame #1 {
            n213 = call "2086组合发送波浪仪.vi"() -> ()  [unwired: 12 in]
          }
          frame #2 {
            n214 = global write "全局1.vi" "2086上传"(FALSE ("2086上传")) -> ()
          }
          frame #3 {
            n215 = call "5001.vi"() -> ()  [unwired: 11 in, 1 out]
          }
        }
      }
    }
    n216 = disable-structure shown="禁用" {
      disable-tunnel: w373 -> [w382 _]
      disable-tunnel: w372 -> [w381 _]
      frame Disabled {
        n217 = stacked-sequence {
          tunnel: w382 -> [w401]
          frame #0 {
            n218 = Get Date/Time In Seconds() -> (seconds since 1Jan1904=w416:timestamp)
            n219 = Get Date/Time String(seconds (now)=w416) -> (time string=w415:string)  [unwired: 2 in, 1 out]
            n220 = Concatenate Strings(w415, "：", w401, "\r\n") -> (w400:string)
            n221 = call <vilib>:"Application Directory.vi"() -> ("Application Directory"=w412:path)
            n222 = Build Path(base path=w412, name or relative path="datasent.txt" ("名称或相对路径")) -> (appended path=w410:path)
            n223 = Open/Create/Replace File(file path (use dialog)=w410, operation (0:open)=T3."open or create" ("操作(0:open)")) -> (refnum out=w408:refnum<file>, error out=w406:errorcluster)  [unwired: 4 in, 1 out]
            n224 = Set File Position(refnum=w408, from (0:start)=enum16{"start", "end", "current"}."end" ("自（0:起始）"), error in=w406) -> (refnum out=w405:refnum<file>, error out=w404:errorcluster)  [unwired: 1 in]
            n225 = Write to Text File(file (use dialog)=w405, text=w400, error in=w404) -> (refnum out=w402:refnum<file>, error out=w403:errorcluster)  [unwired: 1 in, 1 out]
            n226 = Close File(refnum=w402, error in=w403) -> ()  [unwired: 2 out]
            n227 = global write "全局 水样时间.vi" "上传动作"(w400) -> ()
          }
        }
        n228 = stacked-sequence {
          tunnel: w381 -> [_]
          frame #0 {
            n229 = Get Date/Time In Seconds() -> (seconds since 1Jan1904=w399:timestamp)
            n230 = Get Date/Time String(seconds (now)=w399) -> (time string=w398:string)  [unwired: 2 in, 1 out]
            n231 = Concatenate Strings(w398, "：", "Done" ("字符串"), "\r\n") -> (w383:string)
            n232 = call <vilib>:"Application Directory.vi"() -> ("Application Directory"=w395:path)
            n233 = Build Path(base path=w395, name or relative path="datasent.txt" ("名称或相对路径")) -> (appended path=w393:path)
            n234 = Open/Create/Replace File(file path (use dialog)=w393, operation (0:open)=T3."open or create" ("操作(0:open)")) -> (refnum out=w391:refnum<file>, error out=w389:errorcluster)  [unwired: 4 in, 1 out]
            n235 = Set File Position(refnum=w391, from (0:start)=enum16{"start", "end", "current"}."end" ("自（0:起始）"), error in=w389) -> (refnum out=w388:refnum<file>, error out=w387:errorcluster)  [unwired: 1 in]
            n236 = Write to Text File(file (use dialog)=w388, text=w383, error in=w387) -> (refnum out=w385:refnum<file>, error out=w386:errorcluster)  [unwired: 1 in, 1 out]
            n237 = global write "全局 水样时间.vi" "上传动作"(w383) -> ()
            n238 = Close File(refnum=w385, error in=w386) -> ()  [unwired: 2 out]
          }
        }
      }
      frame Enabled {
      }
    }
  }
  n239 = while {
    stop <- FALSE stop-if-true
    # "触发软件自动重启"
    n240 = global read "全局1.vi" "软件自动重启"() -> (w483:dbl)
    n241 = Wait (ms)(milliseconds to wait=u32 1000 ("等待时间（毫秒）")) -> ()  [unwired: 1 out]
    n242 = Greater Or Equal?(x=w483, y=500.0) -> (x >= y?=w481:bool)
    n243 = case shown="True" w481 {
      frame False {
      }
      frame True {
        n244 = flat-sequence {
          frame #0 {
            n245 = call "创建脚本文件.vi"() -> ()  [unwired: 11 in, 1 out]
          }
          frame #1 {
            n246 = global read "断电保存全局.vi" "data名称"() -> (w488:string)
            n247 = Concatenate Strings("data" ("名称或相对路径"), w488, "\\restart.bat" ("字符串")) -> (w486:string)
            n248 = call <vilib>:"Application Directory.vi"() -> ("Application Directory"=w492:path)
            n249 = Build Path(base path=w492, name or relative path=w486) -> (appended path=w493:path)
            n250 = Path To String(path=w493) -> (string=w490:string)
            n251 = call <vilib>:"System Exec.vi"("wait until completion? (T)"=FALSE, "command line"=w490) -> ()  [unwired: 6 in, 4 out]
          }
          frame #2 {
            n252 = global write "全局1.vi" "软件自动重启"(0.0 ("软件自动重启")) -> ()
          }
        }
      }
    }
  }
  n253 = while {
    stop <- FALSE stop-if-true
    # "数据重发"
    n254 = global read "断电保存全局.vi" "每日自动重发"() -> (w496:bool)
    n255 = case shown="False" w496 {
      frame False {
        # "自动重发水样数据"
        n256 = Get Date/Time In Seconds() -> (seconds since 1Jan1904=w499:timestamp)
        n257 = Seconds To Date/Time(time stamp (now)=w499) -> (date time rec=w506:T2)  [unwired: 1 in]
        n258 = Unbundle By Name(w506) -> ("天数（周）"=w511:i32, "时"=w502:i32, "分"=w510:i32)
        n259 = global read "断电保存全局.vi" "重发日期"() -> (w501:T5)
        n260 = global read "断电保存全局.vi" "重发时间"() -> (w500:T6)
        n261 = Equal?(x=w511, y=w501) -> (x = y?=w509:bool)
        n262 = Equal?(x=w502, y=w500) -> (x = y?=w508:bool)
        n263 = Equal?(x=10, y=w510) -> (x = y?=w507:bool)
        n264 = Compound Arithmetic op=AND ("复合运算")(w509, w508, w507) -> (w505:bool)
        n265 = call <vilib>:"Boolean Crossing PtByPt.vi"("direction"=enum16{"either", "false-true", "true-false"}."false-true", "input"=w505) -> ("crossing"=w504:bool)  [unwired: 1 in]
        n266 = case shown="True" w504 {
          tunnel: w499 -> [_ w513]
          frame False {
          }
          frame True {
            n267 = global write "断电保存全局.vi" "数据重发"(TRUE ("数据重发")) -> ()
            n268 = Multiply(x=7.0, y=86400.0) -> (x*y=w515:dbl)
            n269 = Subtract(x=w513, y=w515) -> (x-y=w512:timestamp)
            n270 = Format Date/Time String(time format string (%c)="%Y/%m/%d %H:%M:%S" ("时间格式字符串(%c)"), seconds (now)=w512) -> (date/time string=w517:string)  [unwired: 1 in]
            n271 = global write "断电保存全局.vi" "数据重发时间戳"(w517) -> ()
            n272 = Initialize Array(w517, 76 ("维数大小")) -> (w519:string[])
            n273 = Array To Cluster(array=w519) -> (cluster=w518:T7)
            n274 = global write "全局 水样时间.vi" "水样数据索引"(w518) -> ()
          }
        }
      }
      frame True {
        n275 = Get Date/Time In Seconds() -> (seconds since 1Jan1904=w523:timestamp)
        n276 = Seconds To Date/Time(time stamp (now)=w523) -> (date time rec=w530:T2)  [unwired: 1 in]
        n277 = global read "断电保存全局.vi" "重发时间"() -> (w525:T6)
        n278 = Unbundle By Name(w530) -> ("时"=w526:i32, "分"=w533:i32)
        n279 = Equal?(x=w526, y=w525) -> (x = y?=w532:bool)
        n280 = Equal?(x=10, y=w533) -> (x = y?=w531:bool)
        n281 = Compound Arithmetic op=AND ("复合运算")(w532, w531) -> (w529:bool)
        n282 = call <vilib>:"Boolean Crossing PtByPt.vi"("direction"=enum16{"either", "false-true", "true-false"}."false-true", "input"=w529) -> ("crossing"=w528:bool)  [unwired: 1 in]
        n283 = case shown="True" w528 {
          tunnel: w523 -> [_ w535]
          frame False {
          }
          frame True {
            n284 = global write "断电保存全局.vi" "数据重发"(TRUE ("数据重发")) -> ()
            n285 = Subtract(x=w535, y=86400.0) -> (x-y=w534:timestamp)
            n286 = Format Date/Time String(time format string (%c)="%Y/%m/%d %H:%M:%S" ("时间格式字符串(%c)"), seconds (now)=w534) -> (date/time string=w537:string)  [unwired: 1 in]
            n287 = global write "断电保存全局.vi" "数据重发时间戳"(w537) -> ()
            n288 = Initialize Array(w537, 76 ("维数大小")) -> (w539:string[])
            n289 = Array To Cluster(array=w539) -> (cluster=w538:T7)
            n290 = global write "全局 水样时间.vi" "水样数据索引"(w538) -> ()
          }
        }
      }
    }
    n291 = Wait (ms)(milliseconds to wait=u32 1000 ("等待时间（毫秒）")) -> ()  [unwired: 1 out]
  }
